vi "Automatic-Approach-Retraction-MCL-2013-04-28-1a-data-storage-1b.vi"() -> ()   [LabVIEW 2012]
uses:
  <vilib>/rvi/eio/common/nirviEmuTemplateMethod_errors.vi
  <vilib>/rvi/Emulation/niFpgaSctlEmulationGetInTimedLoop.vi
  <vilib>/rvi/Emulation/niFpgaSctlEmulationGlobalWrite.vi
  <vilib>/rvi/interface/RandomDataEmulation/nirviRandomDataFPGAFIFO.vi
  <vilib>/rvi/interface/RandomDataEmulation/niFpgaRandomDataHandleErrors.vi
  <vilib>/eio/EIONode/EIONode.xnode
  <vilib>/rvi/DataTransferAndStorage/Container/XNode/niFpgaContainer.xnode
  <vilib>/rvi/interface/RandomDataEmulation/nirviRandomDataFpgaReadWriteTemplate.vi
panel:
  out "Tick Count(Ticks)":u32=3198398528
  in  "Data Acquisition Rate (usec)":u32=500000
  out "Data storage":bool=TRUE
  in  "Safetip Control ON/Off":bool
  out "Start Approach indicator":bool
  in  "safetip time wait":u32 caption="Count(uSec)"
  in  "Safetip retraction":u16
  out "safetip minimum indicator":bool
  out "Data counter":u16
  out "Counter Output":i16
  in  "Initial Position":i16
  in  "phase 1 control":bool
  in  "Manual Control":bool
  in  "Zposition MCL fine 2":i16
  in  "MCL counter 2":u16
  out "Curve indicator":u16
  in  "Number of curves":u16
  out "TF Freq shift":i16
  out "USBS Amplitude":i16
  in  "Timeout FIFO":i32=-1
  in  "Safetip Minimum":i16
  out "Phase 2":bool
  in  "Parameter":i16
  out "Phase 1":bool
  in  "Start Approach":bool
  out "MCL counter in range?":bool
  in  "Wait-tip-before-new-approach (usec)":u32
  in  "Fast Retraction After Cycle":i32
  in  "Wait-tip-before-approach":u32
  in  "Fast Retraction before approach":i32
  in  "Offset for Fast Approach":i16
  in  "Fast Approach (usec)":u32
  out "USBS Phase Signal":i16
  in  "Minimum for Approach Value":i16
  out "digital steps per region":u16
  in  "MCL Divisions":u16
  in  "MCL counter":u16
  in  "Fine Retraction (usec)":u32
  in  "TF at infinity":i16
  out "TF Phase Signal":i16(graph)
  out "Control Signal":i16
  out "MCL Sensor":i16
  in  "Fine Approach (usec)":u32
  in  "Setpoint Fine":i16
  out "Zposition MCL fine":i16
  in  "Initial Height (Fine)":i16=9113
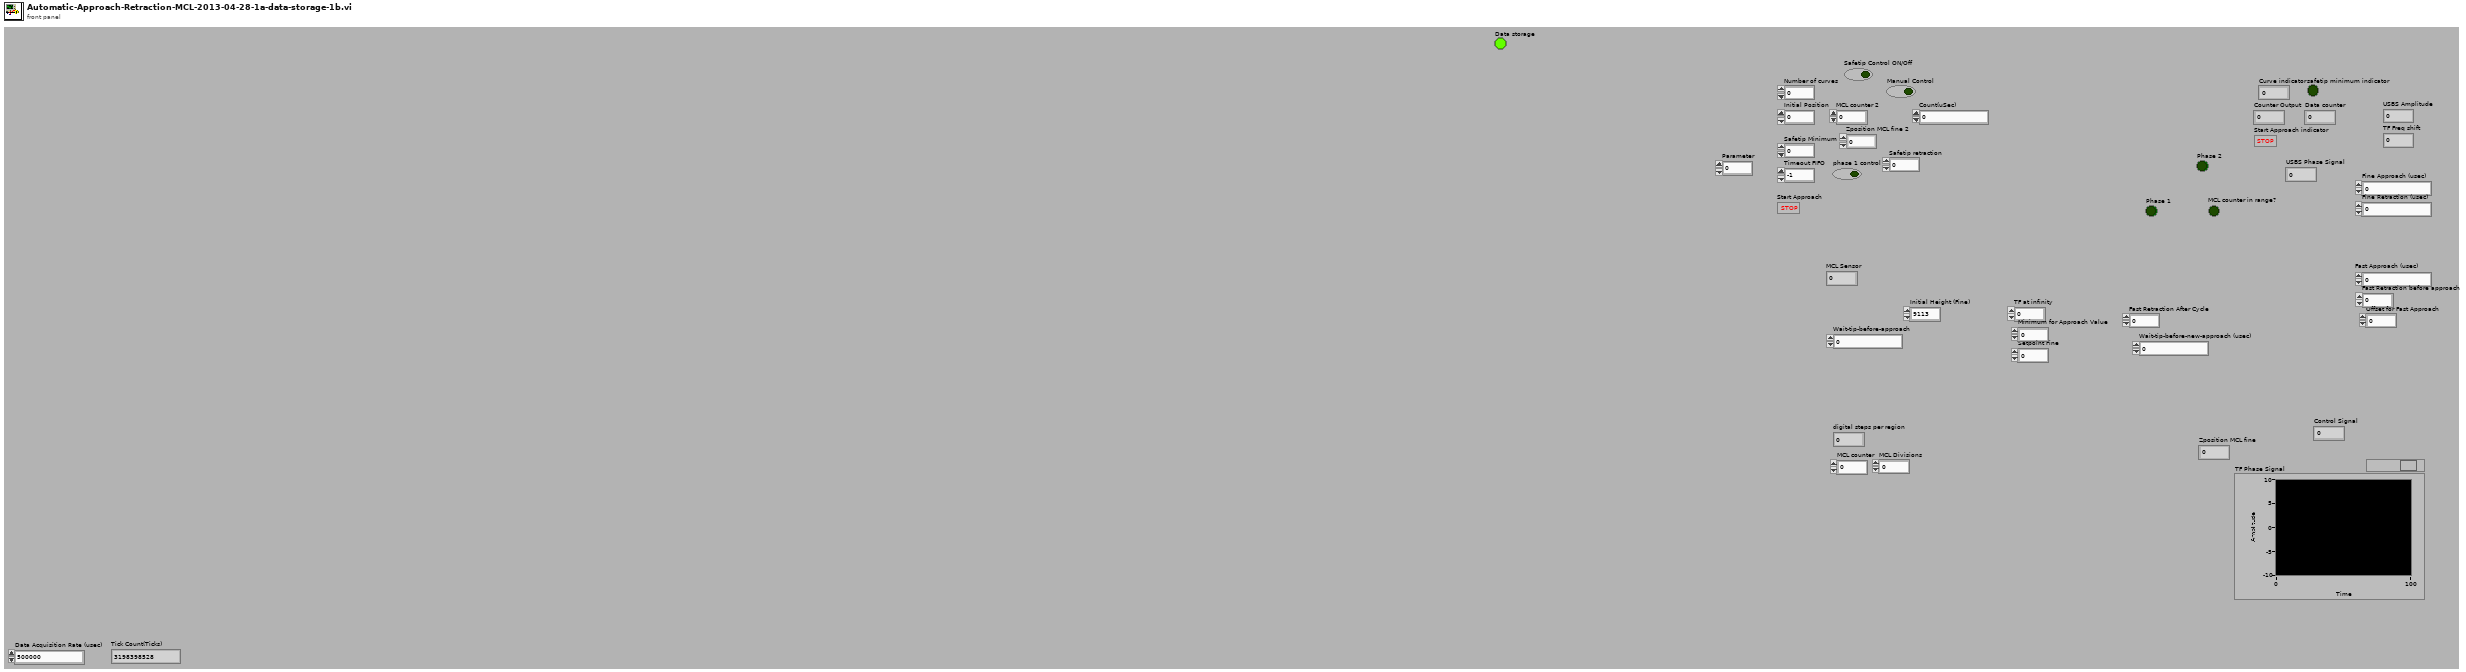
[diagram p1: front panel]
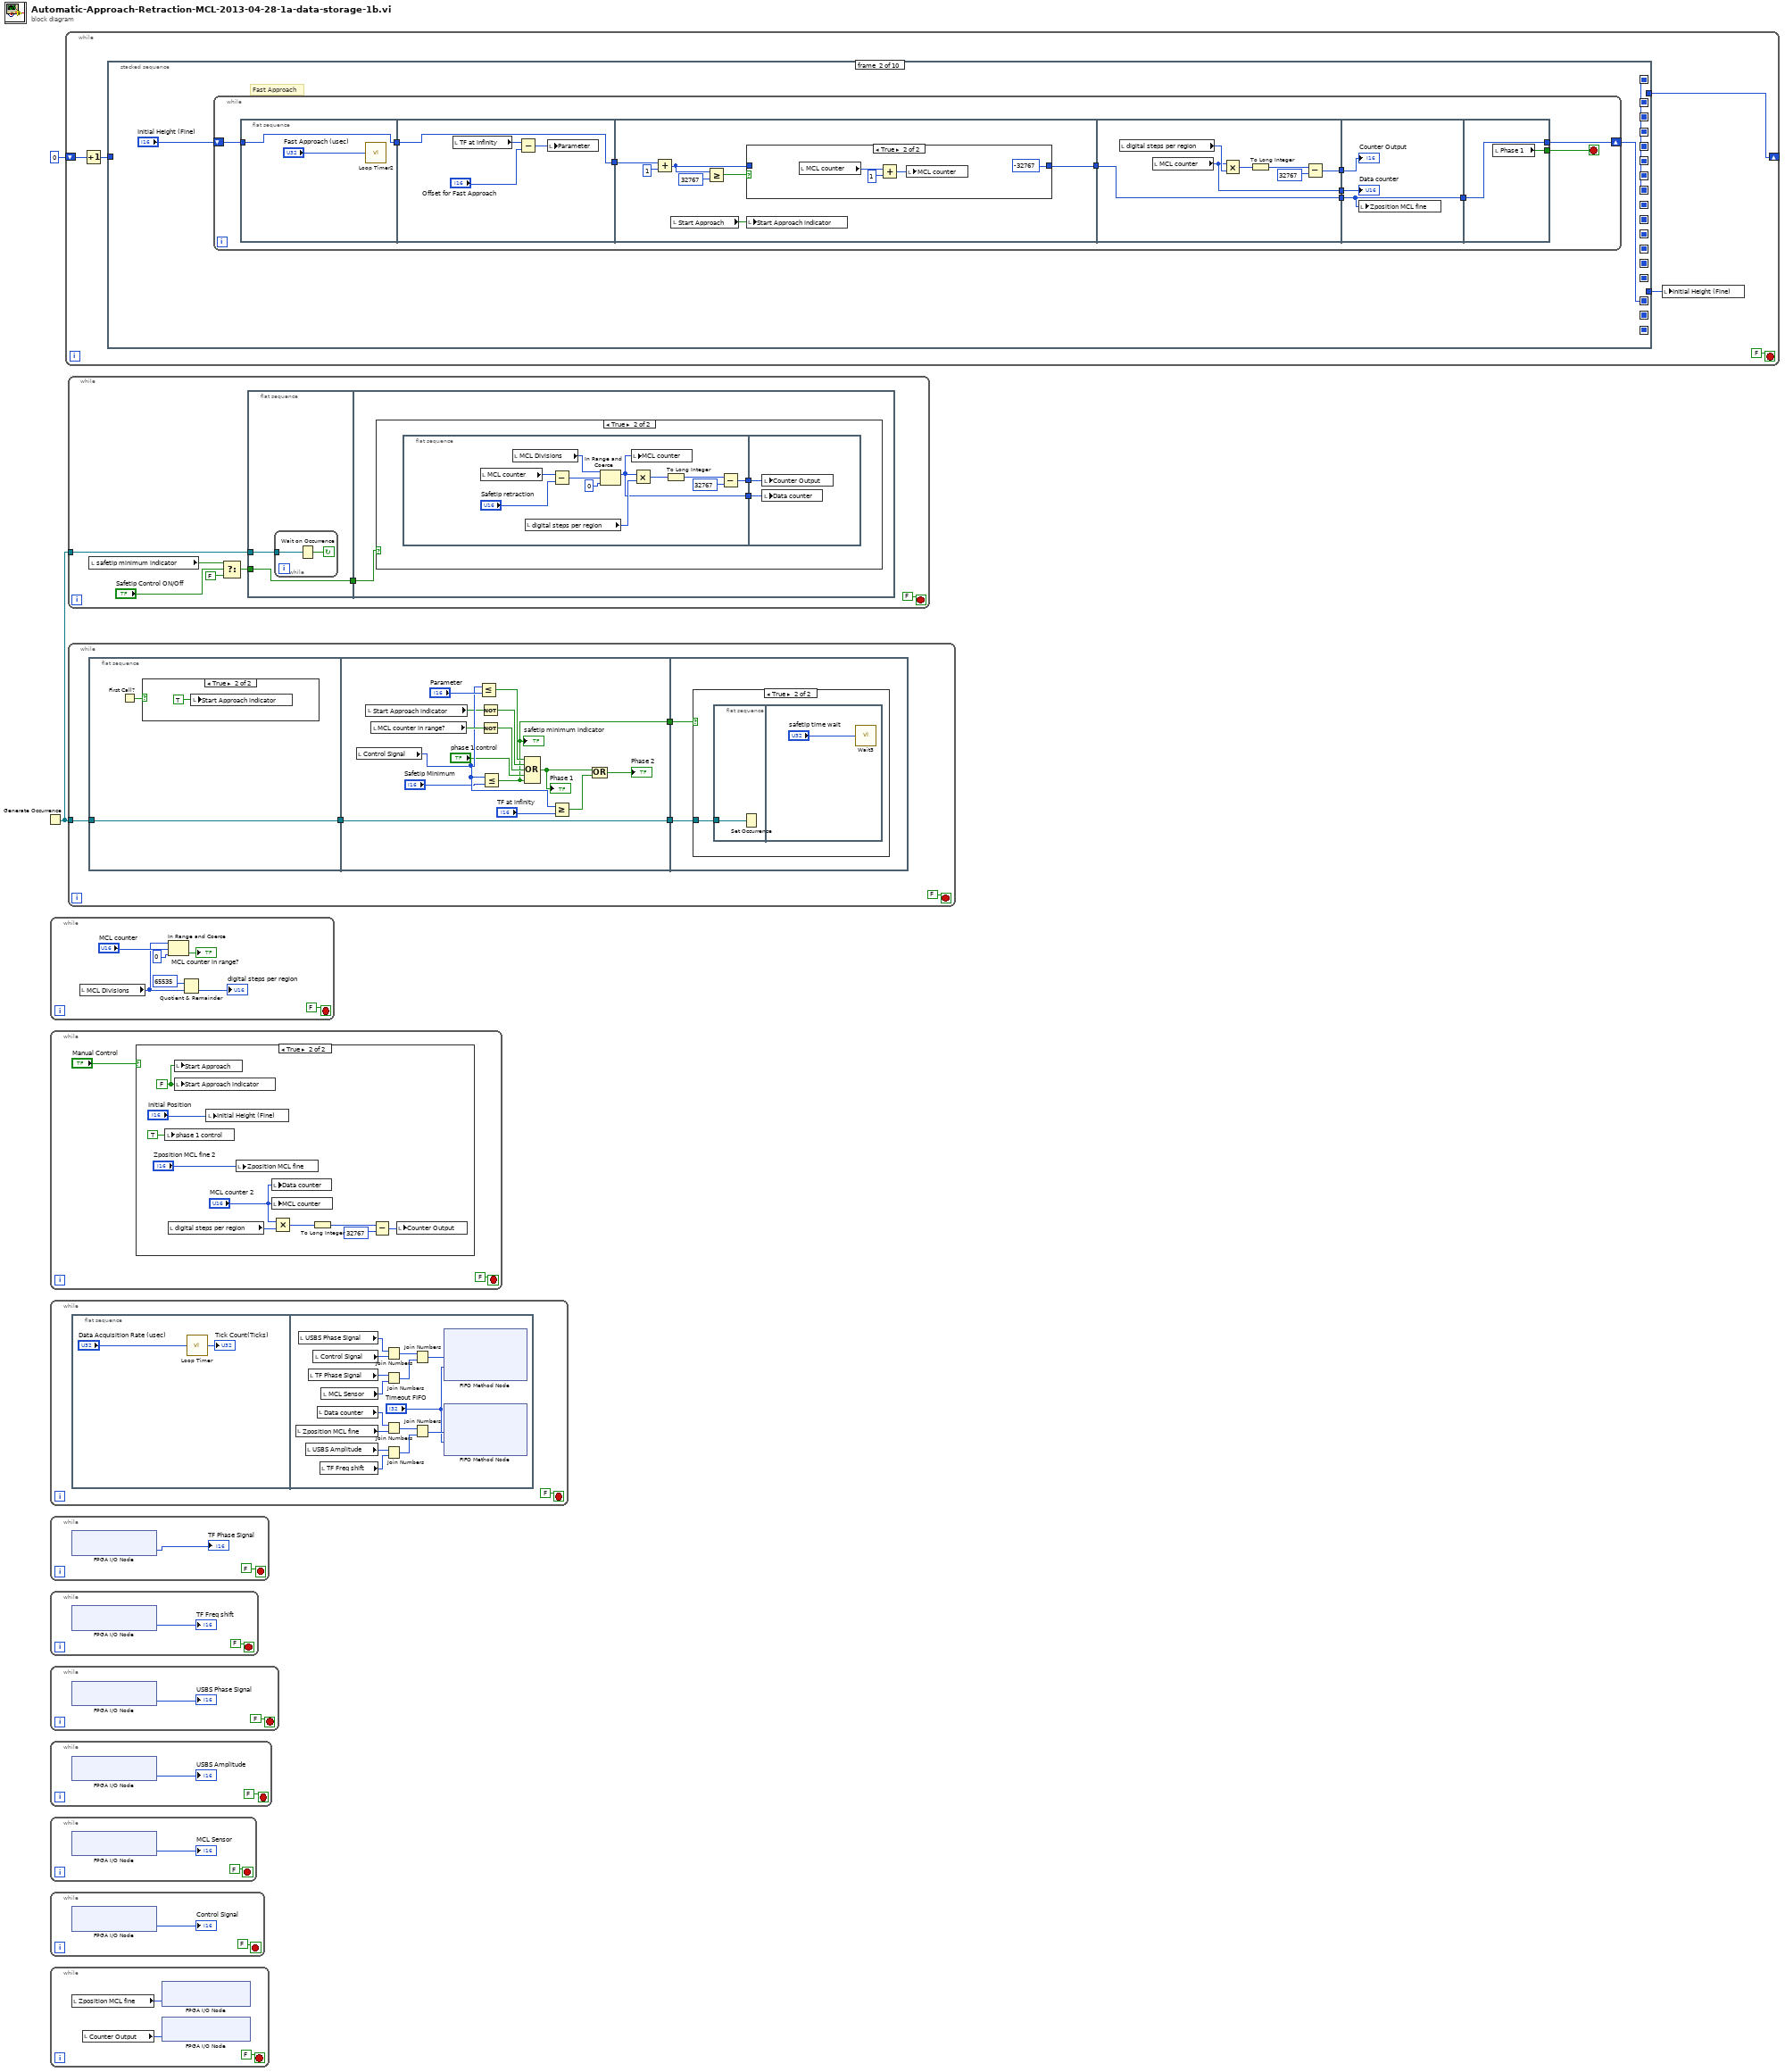
[diagram p0: block diagram]
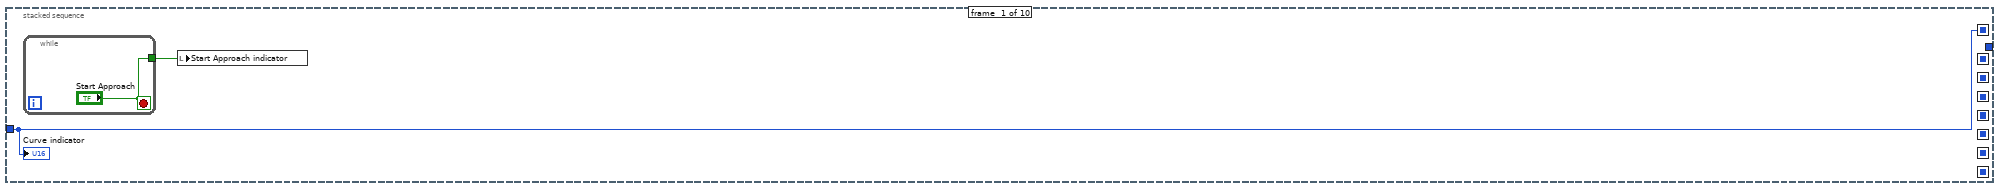
[diagram p6: hidden frame]
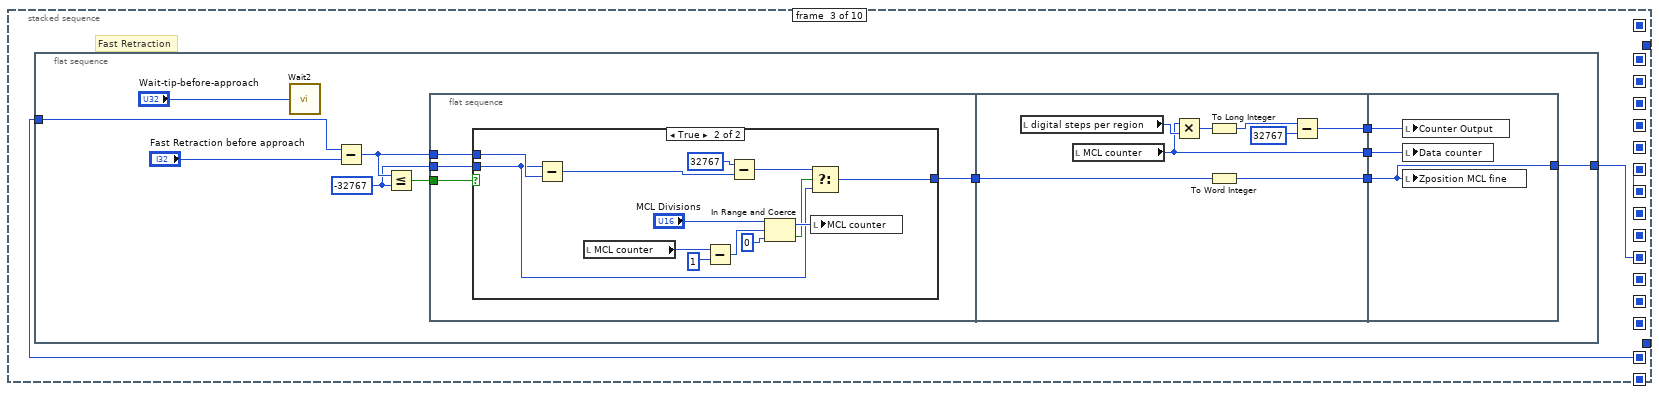
[diagram p8: hidden frame]
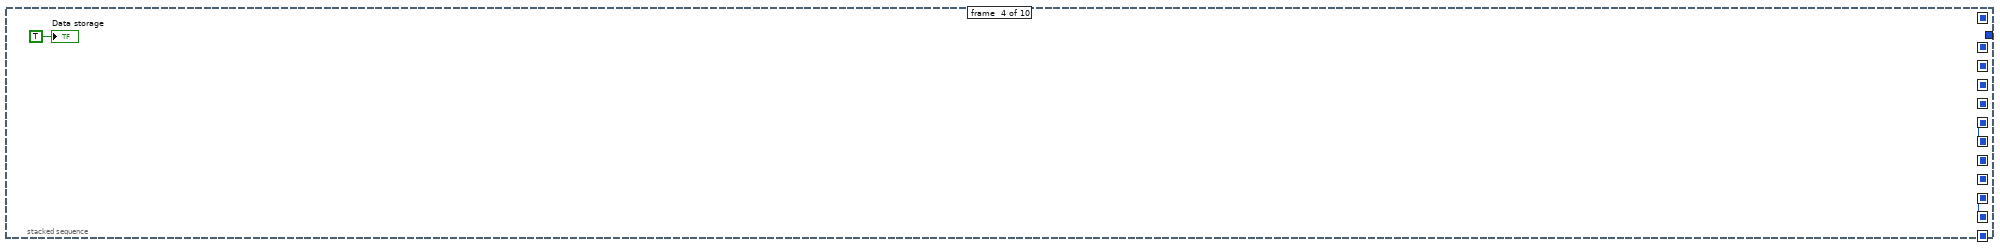
[diagram p10: hidden frame]
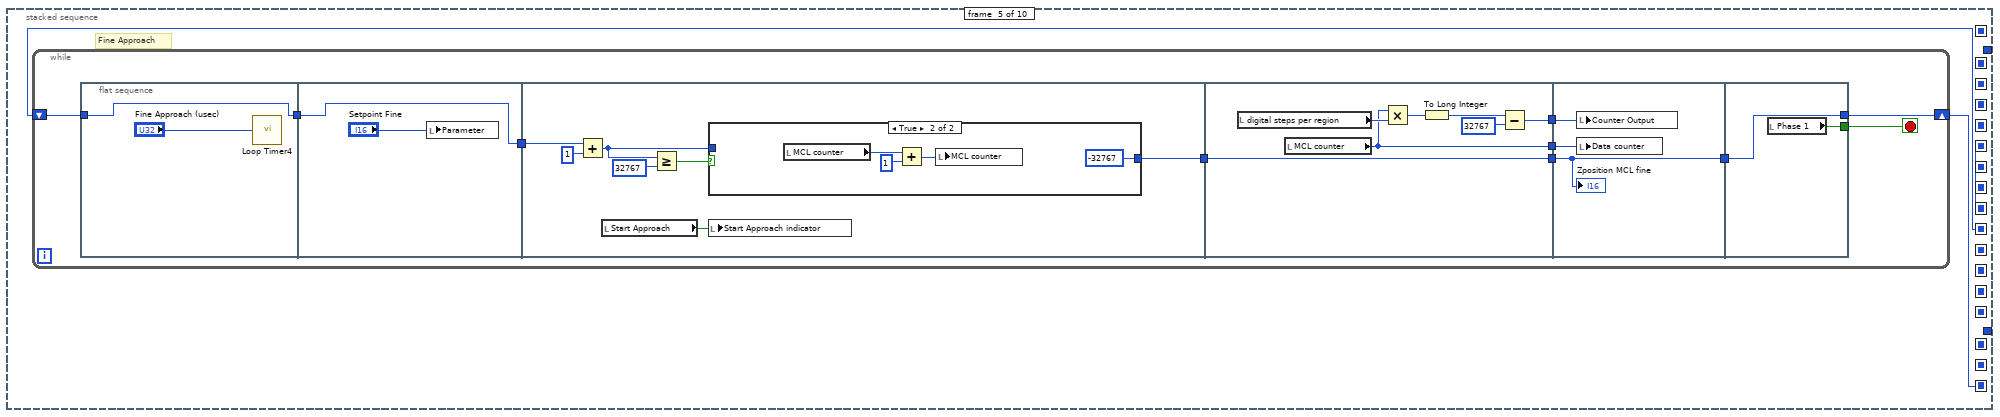
[diagram p11: hidden frame]
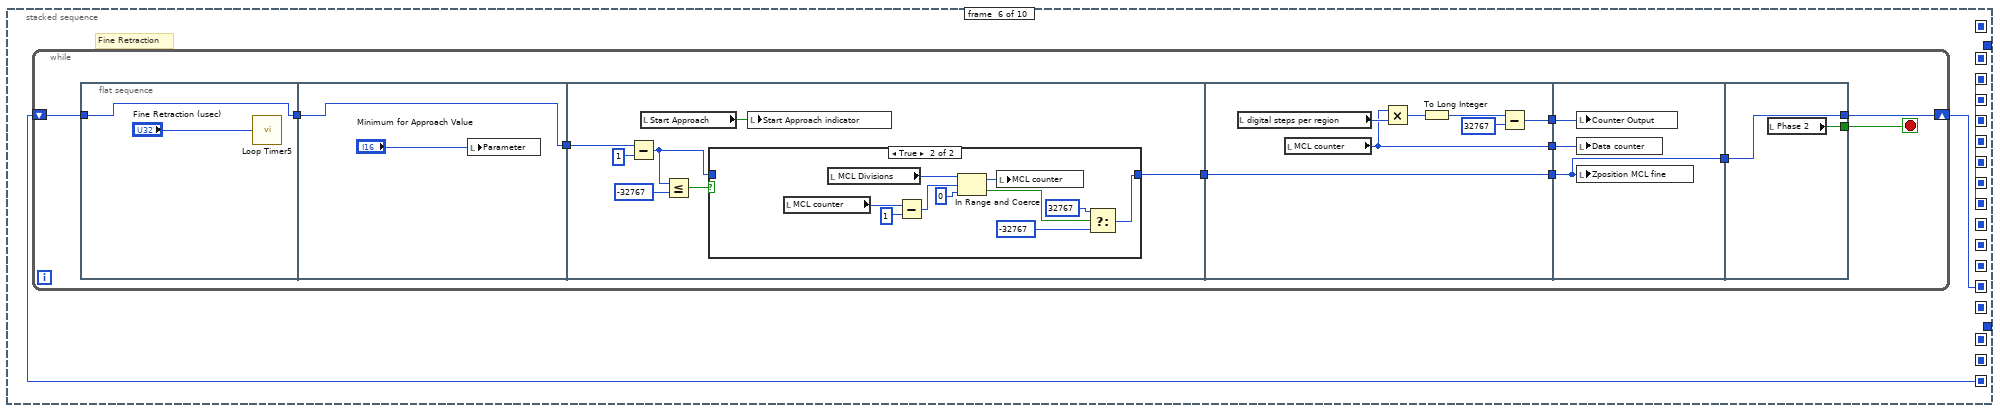
[diagram p13: hidden frame]
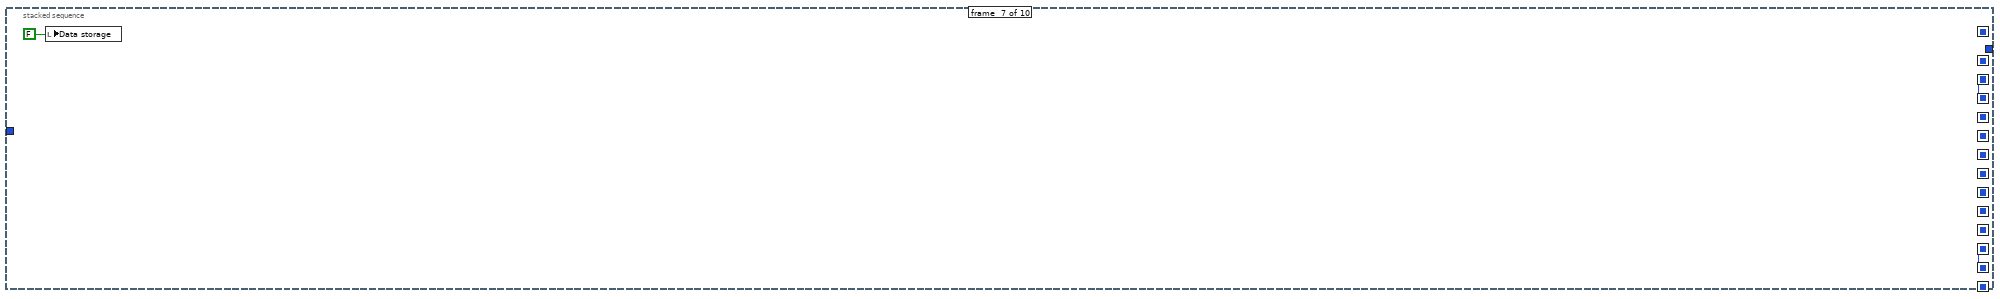
[diagram p15: hidden frame]
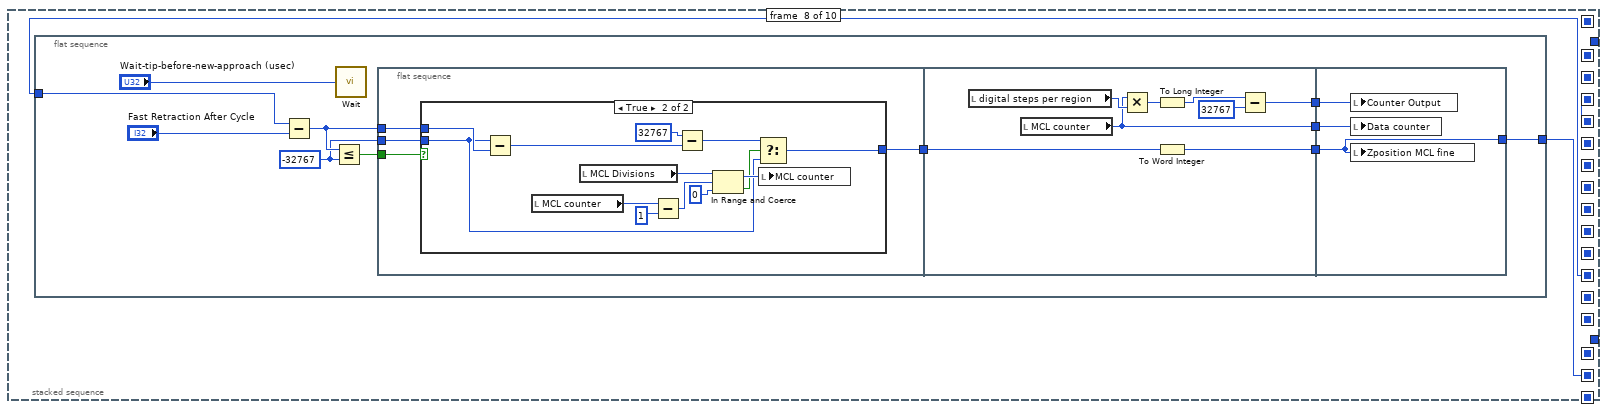
[diagram p16: hidden frame]
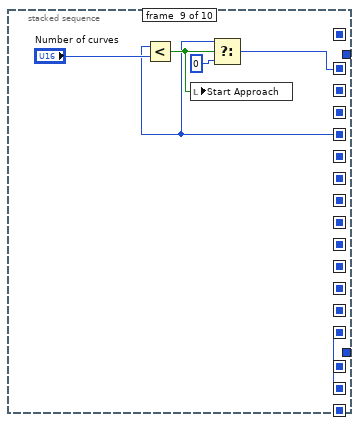
[diagram p18: hidden frame]
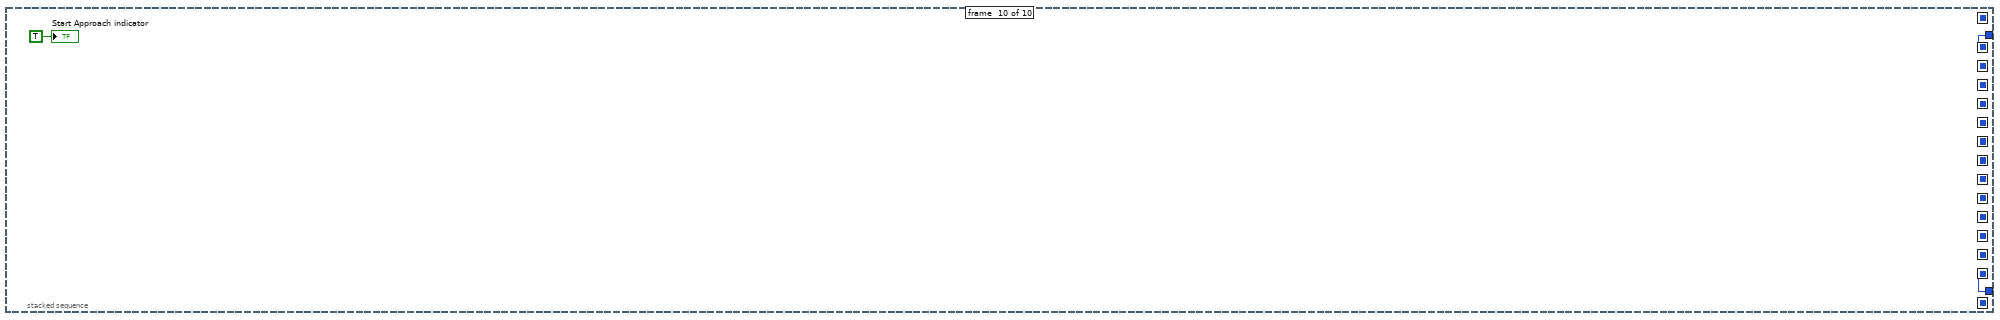
[diagram p19: hidden frame]
diagram:
  n1 = Generate Occurrence() -> (w1:refnum<k4>)
  n2 = while {
    stop <- FALSE stop-if-true
    n3 = local read "MCL Divisions"() -> (w3:u16)
    n4 = In Range and Coerce(upper limit=w3, x="MCL counter", lower limit=u16 0) -> (In Range?=→"MCL counter in range?":bool)  [unwired: 1 out]
    n5 = Quotient & Remainder(x=65535, y=w3) -> (floor(x/y)=→"digital steps per region":i32)  [unwired: 1 out]
  }
  n6 = while {
    stop <- FALSE stop-if-true
    n7 = case shown="True" "Manual Control" {
      frame False {
      }
      frame True {
        w12 = FALSE ("Start Approach")
        n8 = local write "phase 1 control"(TRUE ("phase 1 control")) -> ()
        n9 = local read "digital steps per region"() -> (w18:u16)
        n10 = local write "Start Approach"(w12) -> ()
        n11 = local write "Start Approach indicator"(w12) -> ()
        n12 = local write "Initial Height (Fine)"("Initial Position") -> ()
        n13 = local write "Zposition MCL fine"("Zposition MCL fine 2") -> ()
        n14 = local write "Data counter"("MCL counter 2") -> ()
        n15 = local write "MCL counter"("MCL counter 2") -> ()
        n16 = Multiply(x="MCL counter 2", y=w18) -> (x*y=w14:u16)
        n17 = To Long Integer(number=w14) -> (32bit integer=w13:i32)
        n18 = Subtract(x=w13, y=32767) -> (x-y=w16:i32)
        n19 = local write "Counter Output"(w16) -> ()
      }
    }
  }
  n20 = while {
    stop <- FALSE stop-if-true
    n21 = flat-sequence {
      frame #0 {
        n22 = call "Loop Timer"("Count(Ticks)"="Data Acquisition Rate (usec)") -> ("Tick Count(Ticks)"=→"Tick Count(Ticks)":u32)
      }
      frame #1 {
        n23 = local read "Zposition MCL fine"() -> (w35:i16)
        n24 = local read "USBS Phase Signal"() -> (w30:i16)
        n25 = local read "USBS Amplitude"() -> (w26:i16)
        n26 = local read "TF Phase Signal"() -> (w28:i16)
        n27 = local read "Control Signal"() -> (w29:i16)
        n28 = local read "Data counter"() -> (w36:u16)
        n29 = local read "TF Freq shift"() -> (w25:i16)
        n30 = local read "MCL Sensor"() -> (w27:i16)
        n31 = Join Numbers(hi=w30, lo=w29) -> ((hi.lo)=w38:u32)
        n32 = Join Numbers(hi=w28, lo=w27) -> ((hi.lo)=w39:u32)
        n33 = Join Numbers(hi=w36, lo=w35) -> ((hi.lo)=w33:u32)
        n34 = Join Numbers(hi=w26, lo=w25) -> ((hi.lo)=w34:u32)
        n35 = Join Numbers(hi=w38, lo=w39) -> ((hi.lo)=w37:u64)
        n36 = Join Numbers(hi=w33, lo=w34) -> ((hi.lo)=w32:u64)
        n37 = xnode ("FIFO Method Node")("Element"=w37, "Timeout"="Timeout FIFO") -> ()  [unwired: 1 in, 2 out]
        n38 = xnode ("FIFO Method Node")("Element"=w32, "Timeout"="Timeout FIFO") -> ()  [unwired: 1 in, 2 out]
      }
    }
  }
  n39 = while {
    stop <- FALSE stop-if-true
    n40 = xnode "FPGA I/O Node"() -> ("Connector0/AI1"=→"TF Phase Signal":i16)  [unwired: 1 in, 1 out]
  }
  n41 = while {
    stop <- FALSE stop-if-true
    n42 = xnode "FPGA I/O Node"() -> ("Connector0/AI2"=→"TF Freq shift":i16)  [unwired: 1 in, 1 out]
  }
  n43 = while {
    stop <- FALSE stop-if-true
    n44 = xnode "FPGA I/O Node"() -> ("Connector0/AI4"=→"USBS Phase Signal":i16)  [unwired: 1 in, 1 out]
  }
  n45 = while {
    stop <- FALSE stop-if-true
    n46 = xnode "FPGA I/O Node"() -> ("Connector0/AI5"=→"USBS Amplitude":i16)  [unwired: 1 in, 1 out]
  }
  n47 = while {
    stop <- FALSE stop-if-true
    n48 = xnode "FPGA I/O Node"() -> ("Connector0/AI6"=→"MCL Sensor":i16)  [unwired: 1 in, 1 out]
  }
  n49 = while {
    stop <- FALSE stop-if-true
    n50 = xnode "FPGA I/O Node"() -> ("Connector0/AI7"=→"Control Signal":i16)  [unwired: 1 in, 1 out]
  }
  n51 = while {
    stop <- FALSE stop-if-true
    n52 = local read "Zposition MCL fine"() -> (w53:i16)
    n53 = local read "Counter Output"() -> (w52:i16)
    n54 = xnode "FPGA I/O Node"("Connector0/AO7"=w53) -> ()  [unwired: 1 in, 1 out]
    n55 = xnode "FPGA I/O Node"("Connector0/AO2"=w52) -> ()  [unwired: 1 in, 1 out]
  }
  n56 = while {
    shift-right: [w56] -> _
    shift-left: u16 0 ("t") -> [w55]
    stop <- FALSE stop-if-true
    n57 = Increment(x=w55) -> (x+1=w57:u16)
    n58 = stacked-sequence {
      seq-local: [w61 _ _ _ _ _ _ _ _ _] -> [_ w64 _ _ _ _ _ _ _ _]
      seq-local: [_ w65 _ _ _ _ _ _ _ _] -> [_ _ w108 _ _ _ _ _ _ _]
      seq-local: [_ w64 _ _ _ _ _ _ _ _] -> [_ _ w106 _ _ _ _ _ _ _]
      seq-local: [_ _ w107 _ _ _ _ _ _ _] -> [_ _ _ w151 _ _ _ _ _ _]
      seq-local: [_ _ w106 _ _ _ _ _ _ _] -> [_ _ _ w150 _ _ _ _ _ _]
      seq-local: [_ _ _ w151 _ _ _ _ _ _] -> [_ _ _ _ w154 _ _ _ _ _]
      seq-local: [_ _ _ w150 _ _ _ _ _ _] -> [_ _ _ _ w152 _ _ _ _ _]
      seq-local: [_ _ _ _ w153 _ _ _ _ _] -> [_ _ _ _ _ w195 _ _ _ _]
      seq-local: [_ _ _ _ w152 _ _ _ _ _] -> [_ _ _ _ _ w193 _ _ _ _]
      seq-local: [_ _ _ _ _ w194 _ _ _ _] -> [_ _ _ _ _ _ w242 _ _ _]
      seq-local: [_ _ _ _ _ w193 _ _ _ _] -> [_ _ _ _ _ _ w241 _ _ _]
      seq-local: [_ _ _ _ _ _ w242 _ _ _] -> [_ _ _ _ _ _ _ w245 _ _]
      seq-local: [_ _ _ _ _ _ w241 _ _ _] -> [_ _ _ _ _ _ _ w243 _ _]
      seq-local: [_ _ _ _ _ _ _ w244 _ _] -> [_ _ _ _ _ _ _ _ w291 _]
      seq-local: [_ _ _ _ _ _ _ w243 _ _] -> [_ _ _ _ _ _ _ _ w286 _]
      seq-local: [_ _ _ _ _ _ _ _ w291 _] -> [_ _ _ _ _ _ _ _ _ w294]
      seq-local: [_ _ _ _ _ _ _ _ w287 _] -> [_ _ _ _ _ _ _ _ _ w293]
      tunnel: w57 -> [w61 _ _ _ _ _ _ _ _ _]
      tunnel: [_ _ _ _ _ _ _ _ _ w294] -> w59
      tunnel: [_ _ _ _ _ _ _ _ _ w293] -> w56
      frame #0 {
        n59 = while {
          tunnel: ["Start Approach"] -> w60
          stop <- "Start Approach" stop-if-true
        }
        n60 = local write "Start Approach indicator"(w60) -> ()
        "Curve indicator" <- w61
      }
      frame #1 {
        # "Fast Approach"
        n61 = while {
          shift-right: [w74] -> w65
          shift-left: "Initial Height (Fine)" -> [w75]
          stop <- w70 stop-if-true
          n62 = flat-sequence {
            tunnel: w75 -> [w77]
            tunnel: [w77] -> w72
            tunnel: [w81] -> w73
            tunnel: w72 -> [w81]
            tunnel: [w87] -> w69
            tunnel: w73 -> [w88]
            tunnel: w69 -> [w100]
            tunnel: [w100] -> w68
            tunnel: [w97] -> w67
            tunnel: [w96] -> w66
            tunnel: w68 -> [w103]
            tunnel: [w103] -> w71
            tunnel: w67 -> [w102]
            tunnel: w66 -> [w101]
            tunnel: [w105] -> w74
            tunnel: w71 -> [w105]
            tunnel: [w104] -> w70
            frame #0 {
              n63 = call "Loop Timer2"("Count(uSec)"="Fast Approach (usec)") -> ()  [unwired: 1 out]
            }
            frame #1 {
              n64 = local read "TF at infinity"() -> (w78:i16)
              n65 = Subtract(x=w78, y="Offset for Fast Approach") -> (x-y=w80:i16)
              n66 = local write "Parameter"(w80) -> ()
            }
            frame #2 {
              n67 = Add(x=w88, y=i16 1) -> (x+y=w83:i16)
              n68 = local read "Start Approach"() -> (w82:bool)
              n69 = Greater Or Equal?(x=w83, y=i16 32767) -> (x >= y?=w84:bool)
              n70 = case shown="True" w84 {
                tunnel: [w89 i16 -32767] -> w87
                tunnel: w83 -> [w89 _]
                frame False {
                }
                frame True {
                  n71 = local read "MCL counter"() -> (w91:u16)
                  n72 = Add(x=w91, y=u16 1) -> (x+y=w90:u16)
                  n73 = local write "MCL counter"(w90) -> ()
                }
              }
              n74 = local write "Start Approach indicator"(w82) -> ()
            }
            frame #3 {
              n75 = local read "digital steps per region"() -> (w99:u16)
              n76 = local read "MCL counter"() -> (w96:u16)
              n77 = Multiply(x=w96, y=w99) -> (x*y=w95:u16)
              n78 = To Long Integer(number=w95) -> (32bit integer=w94:i32)
              n79 = Subtract(x=w94, y=32767) -> (x-y=w97:i32)
            }
            frame #4 {
              n80 = local write "Zposition MCL fine"(w103) -> ()
              "Counter Output" <- w102
              "Data counter" <- w101
            }
            frame #5 {
              n81 = local read "Phase 1"() -> (w104:bool)
            }
          }
        }
      }
      frame #2 {
        # "Fast Retraction"
        n82 = flat-sequence {
          tunnel: [w115] -> w107
          tunnel: w108 -> [w116]
          frame #0 {
            w113 = -32767 ("y")
            n83 = call "Wait2"("Count(uSec)"="Wait-tip-before-approach") -> ()  [unwired: 1 out]
            n84 = Subtract(x=w116, y="Fast Retraction before approach") -> (x-y=w118:i32)
            n85 = Less Or Equal?(x=w118, y=w113) -> (x <= y?=w119:bool)
            n86 = flat-sequence {
              tunnel: w119 -> [w123]
              tunnel: w118 -> [w122]
              tunnel: w113 -> [w120]
              tunnel: [w121] -> w112
              tunnel: w112 -> [w141]
              tunnel: [w140] -> w111
              tunnel: [w142] -> w110
              tunnel: [w143] -> w109
              tunnel: [w148] -> w115
              tunnel: w111 -> [w148]
              tunnel: w110 -> [w147]
              tunnel: w109 -> [w146]
              frame #0 {
                n87 = case shown="True" w123 {
                  tunnel: w122 -> [w124 w134]
                  tunnel: [w124 w126] -> w121
                  tunnel: w120 -> [_ w125]
                  frame False {
                  }
                  frame True {
                    n88 = Subtract(x=w125, y=w134) -> (x-y=w133:i32)
                    n89 = local read "MCL counter"() -> (w137:u16)
                    n90 = Subtract(x=w137, y=u16 1) -> (x-y=w130:u16)
                    n91 = Subtract(x=32767, y=w133) -> (x-y=w127:i32)
                    n92 = In Range and Coerce(upper limit="MCL Divisions", x=w130, lower limit=u16 0 ("upper limit")) -> (coerced(x)=w129:u16, In Range?=w128:bool)
                    n93 = Select(t=w127, s=w128, f=w125) -> (s? t:f=w126:i32)
                    n94 = local write "MCL counter"(w129) -> ()
                  }
                }
              }
              frame #1 {
                n95 = local read "digital steps per region"() -> (w145:u16)
                n96 = local read "MCL counter"() -> (w142:u16)
                n97 = Multiply(x=w142, y=w145) -> (x*y=w139:u16)
                n98 = To Long Integer(number=w139) -> (32bit integer=w138:i32)
                n99 = To Word Integer(number=w141) -> (16bit integer=w140:i16)
                n100 = Subtract(x=w138, y=32767) -> (x-y=w143:i32)
              }
              frame #2 {
                n101 = local write "Counter Output"(w146) -> ()
                n102 = local write "Data counter"(w147) -> ()
                n103 = local write "Zposition MCL fine"(w148) -> ()
              }
            }
          }
        }
      }
      frame #3 {
        "Data storage" <- TRUE
      }
      frame #4 {
        # "Fine Approach"
        n104 = while {
          shift-right: [w163] -> w153
          shift-left: w154 -> [w164]
          stop <- w155 stop-if-true
          n105 = flat-sequence {
            tunnel: w164 -> [w166]
            tunnel: [w166] -> w161
            tunnel: [w168] -> w162
            tunnel: w161 -> [w168]
            tunnel: [w174] -> w160
            tunnel: w162 -> [w175]
            tunnel: w160 -> [w187]
            tunnel: [w187] -> w159
            tunnel: [w184] -> w158
            tunnel: [w183] -> w157
            tunnel: w159 -> [w188]
            tunnel: w158 -> [w190]
            tunnel: w157 -> [w189]
            tunnel: [w188] -> w156
            tunnel: [w192] -> w163
            tunnel: w156 -> [w192]
            tunnel: [w191] -> w155
            frame #0 {
              n106 = call "Loop Timer4"("Count(uSec)"="Fine Approach (usec)") -> ()  [unwired: 1 out]
            }
            frame #1 {
              n107 = local write "Parameter"("Setpoint Fine") -> ()
            }
            frame #2 {
              n108 = Add(x=w175, y=i16 1) -> (x+y=w170:i16)
              n109 = local read "Start Approach"() -> (w169:bool)
              n110 = Greater Or Equal?(x=w170, y=i16 32767) -> (x >= y?=w171:bool)
              n111 = case shown="True" w171 {
                tunnel: [w176 i16 -32767] -> w174
                tunnel: w170 -> [w176 _]
                frame False {
                }
                frame True {
                  n112 = local read "MCL counter"() -> (w177:u16)
                  n113 = Add(x=w177, y=u16 1) -> (x+y=w179:u16)
                  n114 = local write "MCL counter"(w179) -> ()
                }
              }
              n115 = local write "Start Approach indicator"(w169) -> ()
            }
            frame #3 {
              n116 = local read "digital steps per region"() -> (w186:u16)
              n117 = local read "MCL counter"() -> (w183:u16)
              n118 = Multiply(x=w183, y=w186) -> (x*y=w182:u16)
              n119 = To Long Integer(number=w182) -> (32bit integer=w181:i32)
              n120 = Subtract(x=w181, y=32767) -> (x-y=w184:i32)
            }
            frame #4 {
              n121 = local write "Counter Output"(w190) -> ()
              n122 = local write "Data counter"(w189) -> ()
              "Zposition MCL fine" <- w188
            }
            frame #5 {
              n123 = local read "Phase 1"() -> (w191:bool)
            }
          }
        }
      }
      frame #5 {
        # "Fine Retraction"
        n124 = while {
          shift-right: [w204] -> w194
          shift-left: w195 -> [w205]
          stop <- w198 stop-if-true
          n125 = flat-sequence {
            tunnel: w205 -> [w207]
            tunnel: [w207] -> w201
            tunnel: [w209] -> w202
            tunnel: w201 -> [w209]
            tunnel: [w215] -> w203
            tunnel: w202 -> [w216]
            tunnel: w203 -> [w234]
            tunnel: [w234] -> w200
            tunnel: [w229] -> w197
            tunnel: [w228] -> w196
            tunnel: w200 -> [w235]
            tunnel: [w235] -> w199
            tunnel: w197 -> [w237]
            tunnel: w196 -> [w236]
            tunnel: [w239] -> w204
            tunnel: w199 -> [w239]
            tunnel: [w238] -> w198
            frame #0 {
              n126 = call "Loop Timer5"("Count(uSec)"="Fine Retraction (usec)") -> ()  [unwired: 1 out]
            }
            frame #1 {
              n127 = local write "Parameter"("Minimum for Approach Value") -> ()
            }
            frame #2 {
              n128 = Subtract(x=w216, y=i16 1) -> (x-y=w211:i16)
              n129 = local read "Start Approach"() -> (w210:bool)
              n130 = Less Or Equal?(x=w211, y=i16 -32767) -> (x <= y?=w213:bool)
              n131 = case shown="True" w213 {
                tunnel: w211 -> [w217 _]
                tunnel: [w217 w218] -> w215
                frame False {
                }
                frame True {
                  n132 = local read "MCL counter"() -> (w227:u16)
                  n133 = local read "MCL Divisions"() -> (w225:u16)
                  n134 = Subtract(x=w227, y=u16 1) -> (x-y=w223:u16)
                  n135 = In Range and Coerce(upper limit=w225, x=w223, lower limit=u16 0) -> (coerced(x)=w222:u16, In Range?=w221:bool)
                  n136 = local write "MCL counter"(w222) -> ()
                  n137 = Select(t=i16 32767, s=w221, f=i16 -32767) -> (s? t:f=w218:i16)
                }
              }
              n138 = local write "Start Approach indicator"(w210) -> ()
            }
            frame #3 {
              n139 = local read "digital steps per region"() -> (w233:u16)
              n140 = local read "MCL counter"() -> (w229:u16)
              n141 = Multiply(x=w229, y=w233) -> (x*y=w231:u16)
              n142 = To Long Integer(number=w231) -> (32bit integer=w230:i32)
              n143 = Subtract(x=w230, y=32767) -> (x-y=w228:i32)
            }
            frame #4 {
              n144 = local write "Counter Output"(w236) -> ()
              n145 = local write "Data counter"(w237) -> ()
              n146 = local write "Zposition MCL fine"(w235) -> ()
            }
            frame #5 {
              n147 = local read "Phase 2"() -> (w238:bool)
            }
          }
        }
      }
      frame #6 {
        n148 = local write "Data storage"(FALSE ("Data storage")) -> ()
      }
      frame #7 {
        n149 = flat-sequence {
          tunnel: [w252] -> w244
          tunnel: w245 -> [w253]
          frame #0 {
            w250 = -32767 ("y")
            n150 = Subtract(x=w253, y="Fast Retraction After Cycle") -> (x-y=w256:i32)
            n151 = Less Or Equal?(x=w256, y=w250) -> (x <= y?=w255:bool)
            n152 = call "Wait"("Count(uSec)"="Wait-tip-before-new-approach (usec)") -> ()  [unwired: 1 out]
            n153 = flat-sequence {
              tunnel: w256 -> [w260]
              tunnel: w255 -> [w259]
              tunnel: w250 -> [w257]
              tunnel: [w258] -> w249
              tunnel: w249 -> [w278]
              tunnel: [w277] -> w248
              tunnel: [w280] -> w247
              tunnel: [w279] -> w246
              tunnel: [w284] -> w252
              tunnel: w248 -> [w284]
              tunnel: w247 -> [w285]
              tunnel: w246 -> [w283]
              frame #0 {
                n154 = case shown="True" w259 {
                  tunnel: w260 -> [w261 w272]
                  tunnel: [w261 w262] -> w258
                  tunnel: w257 -> [_ w263]
                  frame False {
                  }
                  frame True {
                    n155 = Subtract(x=w263, y=w272) -> (x-y=w271:i32)
                    n156 = local read "MCL counter"() -> (w274:u16)
                    n157 = local read "MCL Divisions"() -> (w268:u16)
                    n158 = Subtract(x=w274, y=u16 1) -> (x-y=w269:u16)
                    n159 = Subtract(x=32767, y=w271) -> (x-y=w264:i32)
                    n160 = In Range and Coerce(upper limit=w268, x=w269, lower limit=u16 0) -> (coerced(x)=w266:u16, In Range?=w265:bool)
                    n161 = Select(t=w264, s=w265, f=w263) -> (s? t:f=w262:i32)
                    n162 = local write "MCL counter"(w266) -> ()
                  }
                }
              }
              frame #1 {
                n163 = local read "digital steps per region"() -> (w282:u16)
                n164 = local read "MCL counter"() -> (w279:u16)
                n165 = Multiply(x=w279, y=w282) -> (x*y=w276:u16)
                n166 = To Long Integer(number=w276) -> (32bit integer=w275:i32)
                n167 = To Word Integer(number=w278) -> (16bit integer=w277:i16)
                n168 = Subtract(x=w275, y=32767) -> (x-y=w280:i32)
              }
              frame #2 {
                n169 = local write "Counter Output"(w285) -> ()
                n170 = local write "Data counter"(w283) -> ()
                n171 = local write "Zposition MCL fine"(w284) -> ()
              }
            }
          }
        }
      }
      frame #8 {
        n172 = Less?(x=w286, y="Number of curves") -> (x < y?=w289:bool)
        n173 = local write "Start Approach"(w289) -> ()
        n174 = Select(t=w286, s=w289, f=u16 0 ("t")) -> (s? t:f=w287:u16)
      }
      frame #9 {
        "Start Approach indicator" <- TRUE ("Start Approach indicator")
      }
    }
    n175 = local write "Initial Height (Fine)"(w59) -> ()
  }
  n176 = while {
    tunnel: w1 -> [w297]
    stop <- FALSE stop-if-true
    n177 = local read "safetip minimum indicator"() -> (w300:bool)
    n178 = Select(t=w300, s="Safetip Control ON/Off", f=FALSE) -> (s? t:f=w295:bool)
    n179 = flat-sequence {
      tunnel: w297 -> [w303]
      tunnel: [w302] -> w296
      tunnel: w295 -> [w302]
      tunnel: w296 -> [w306]
      frame #0 {
        n180 = while {
          tunnel: w303 -> [w304]
          stop <- w305 continue-if-true
          n181 = Wait on Occurrence(2:w304) -> (0:w305:bool)  [unwired: 2 in]
        }
      }
      frame #1 {
        n182 = case shown="True" w306 {
          frame False {
          }
          frame True {
            n183 = flat-sequence {
              tunnel: [w313] -> w308
              tunnel: [w309] -> w307
              tunnel: w308 -> [w321]
              tunnel: w307 -> [w320]
              frame #0 {
                n184 = local read "MCL counter"() -> (w317:u16)
                n185 = local read "MCL Divisions"() -> (w316:u16)
                n186 = local read "digital steps per region"() -> (w319:u16)
                n187 = Subtract(x=w317, y="Safetip retraction") -> (x-y=w314:u16)
                n188 = In Range and Coerce(upper limit=w316, x=w314, lower limit=u16 0) -> (coerced(x)=w313:u16)  [unwired: 1 out]
                n189 = local write "MCL counter"(w313) -> ()
                n190 = Multiply(x=w313, y=w319) -> (x*y=w312:u16)
                n191 = To Long Integer(number=w312) -> (32bit integer=w311:i32)
                n192 = Subtract(x=w311, y=32767) -> (x-y=w309:i32)
              }
              frame #1 {
                n193 = local write "Counter Output"(w320) -> ()
                n194 = local write "Data counter"(w321) -> ()
              }
            }
          }
        }
      }
    }
  }
  n195 = while {
    tunnel: w1 -> [w324]
    stop <- FALSE stop-if-true
    n196 = flat-sequence {
      tunnel: [w327] -> w325
      tunnel: w324 -> [w327]
      tunnel: [w332] -> w323
      tunnel: w325 -> [w330]
      tunnel: [w330] -> w322
      tunnel: w323 -> [w346]
      tunnel: w322 -> [w345]
      frame #0 {
        n197 = First Call?() -> (First Call?: T/F=w328:bool)
        n198 = case shown="True" w328 {
          frame False {
          }
          frame True {
            n199 = local write "Start Approach indicator"(TRUE ("Start Approach indicator")) -> ()
          }
        }
      }
      frame #1 {
        n200 = local read "Control Signal"() -> (w336:i16)
        n201 = local read "Start Approach indicator"() -> (w331:bool)
        n202 = local read "MCL counter in range?"() -> (w343:bool)
        n203 = Less Or Equal?(x=w336, y="Parameter") -> (x <= y?=w341:bool)
        n204 = Not(x=w331) -> (.not. x?=w342:bool)
        n205 = Not(x=w343) -> (.not. x?=w344:bool)
        n206 = Less Or Equal?(x=w336, y="Safetip Minimum") -> (x <= y?=w332:bool)
        "safetip minimum indicator" <- w332
        n207 = Compound Arithmetic op=OR(w341, w342, w344, "phase 1 control", w332) -> (w333:bool)
        "Phase 1" <- w333
        n208 = Greater Or Equal?(x=w336, y="TF at infinity") -> (x >= y?=w338:bool)
        n209 = Compound Arithmetic op=OR(w333, w338) -> (→"Phase 2":bool)
      }
      frame #2 {
        n210 = case shown="True" w346 {
          tunnel: w345 -> [_ w347]
          frame False {
          }
          frame True {
            n211 = flat-sequence {
              tunnel: w347 -> [w348]
              frame #0 {
                n212 = Set Occurrence(w348) -> ()
              }
              frame #1 {
                n213 = call "Wait3"("Count(uSec)"="safetip time wait") -> ()  [unwired: 1 out]
              }
            }
          }
        }
      }
    }
  }
